vi "Result.Numeric, Array, Convert V2 to Measurement V1 Format.vi"(11 "Num In":T3[](array[typedef]) {"Status" items=["LOG", "PASS", "FAIL", "ERROR"]}) -> (3 "Meas Out":T1[](array[typedef]) {"Status" items=["LOG", "PASS", "FAIL", "ERROR"]})   [LabVIEW 2024]
uses:
  Result.Numeric.ctl
  Result.Limit Type.ctl
  Result.Measurement and Attribute Item Status.ctl
  Result.Measurement Item.ctl
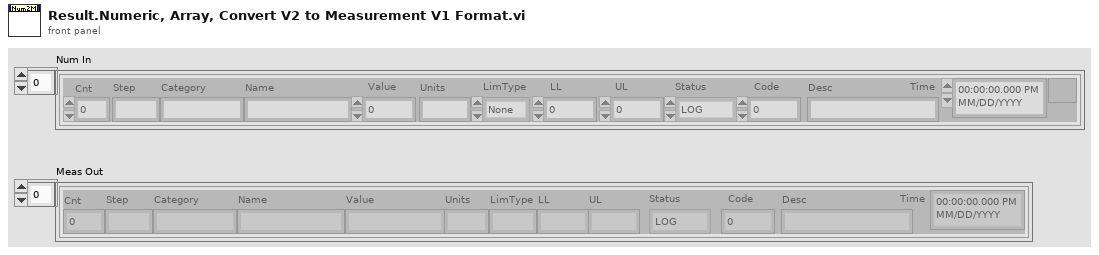
[diagram p1: front panel]
types:
  T1 = typedef "Result.Measurement Item.ctl" = cluster{"Cnt":i32, "Step":string, "Category":string, "Name":string, "Value":string, "Units":string, "LimType":string, "LL":string, "UL":string, "Status":T2, "Code":i32, "Desc":string, "Time":timestamp}
  T2 = typedef "Result.Measurement and Attribute Item Status.ctl" = i32
  T3 = typedef "Result.Numeric.ctl" = cluster{"Cnt":i32, "Step":string, "Category":string, "Name":string, "Value":dbl, "Units":string, "LimType":T4, "LL":dbl, "UL":dbl, "Status":T2, "Code":i32, "Desc":string, "Time":timestamp}
  T4 = typedef "Result.Limit Type.ctl" = enum16{"None", "EQ", "NE", "GT", "LT", "GE", "LE", "GTLT", "GELE", "GELT", "GTLE", "LTGT", "LEGE", "LEGT", "LTGE", "Contains", "NotContains"}
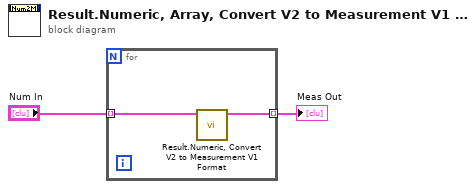
[diagram p0: block diagram]
diagram:
  n1 = for {
    tunnel: "Num In" -> [w4] mode=indexing
    tunnel: [w3] -> w1 mode=indexing
    n2 = call "Result.Numeric, Convert V2 to Measurement V1 Format.vi"("Measurement"=w4) -> ("Meas"=w3:T1)  [unwired: 10 in]
  }
  "Meas Out" <- w1
